vi "reference.vi"(10 "Enum":enum16{"clear", "read", "write"}(ring)=enum."write", 11 "referenceImageIn":i32[][](array[numeric])) -> (3 "referenceImageOut":i32[][](array[numeric]))   [LabVIEW 2016]
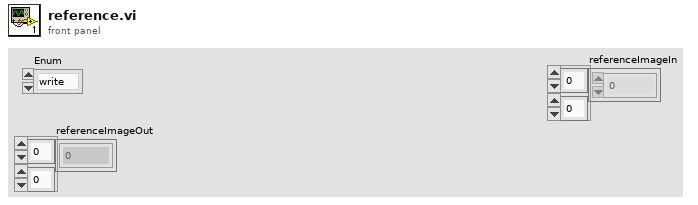
[diagram p1: front panel]
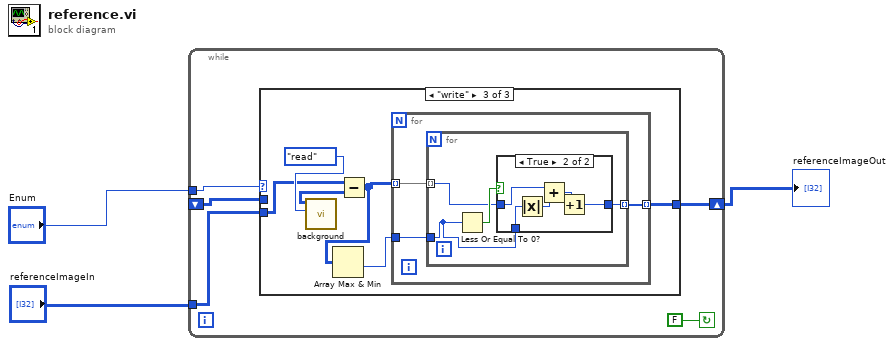
[diagram p0: block diagram]
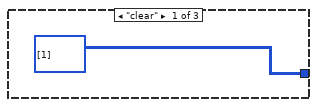
[diagram p2: hidden frame]
diagram:
  n1 = while {
    tunnel: "Enum" -> [w7]
    shift-right: [w6] -> w2
    shift-left: _ -> [w4]
    tunnel: "referenceImageIn" -> [w5]
    stop <- FALSE continue-if-true
    n2 = case shown="\"write\"" w7 {
      tunnel: w5 -> [_ _ w14]
      tunnel: [i32[][] [[1]] ("imageCube") w10 w13] -> w6
      tunnel: w4 -> [_ w10 _]
      frame "clear" {
      }
      frame "read", Default {
      }
      frame "write" {
        n3 = call "background.vi"("Enum"=enum16{"clear", "read", "write"}."read") -> ("backgroundImageOut"=w15:i32[][])  [unwired: 10 in]
        n4 = Subtract(x=w14, y=w15) -> (x-y=w12:i32[][])
        n5 = Array Max & Min(array=w12) -> (min value=w11:i32)  [unwired: 3 out]
        n6 = for {
          tunnel: w12 -> [w19] mode=indexing
          tunnel: [w18] -> w13 mode=indexing
          tunnel: w11 -> [w17]
          n7 = for {
            tunnel: w19 -> [w21] mode=indexing
            tunnel: [w22] -> w18 mode=indexing
            tunnel: w17 -> [w20]
            n8 = Less Or Equal To 0?(x=w20) -> (x <= 0?=w23:bool)
            n9 = case shown="True" w23 {
              tunnel: [w24 w25] -> w22
              tunnel: w21 -> [w24 w29]
              tunnel: w20 -> [_ w26]
              frame False {
              }
              frame True {
                n10 = Absolute Value(x=w26) -> (abs(x)=w27:i32)
                n11 = Add(x=w29, y=w27) -> (x+y=w28:i32)
                n12 = Increment(x=w28) -> (x+1=w25:i32)
              }
            }
          }
        }
      }
    }
  }
  "referenceImageOut" <- w2
